vi "Reset WT300 Integrator.vi"(8 "error in (no error)":errorcluster, 11 "VISA resource name":refnum<visa-resource-name>) -> (0 "error out":errorcluster, 3 "VISA resource name out":refnum<visa-resource-name>)   [LabVIEW 2019, in "Yokogawa WT300 Series.lvlib"]
uses:
  Yokogawa WT300 Series.lvlib
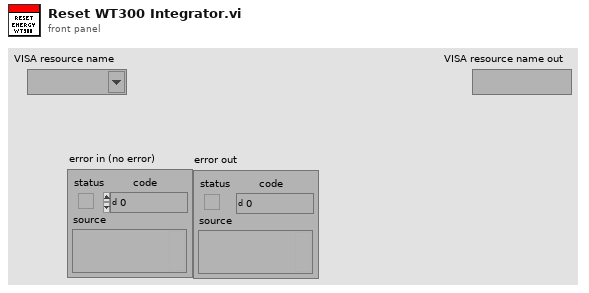
[diagram p1: front panel]
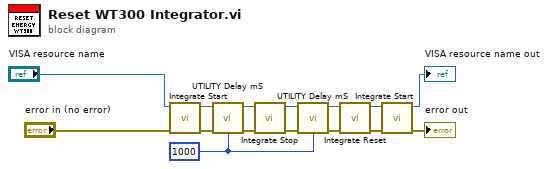
[diagram p0: block diagram]
diagram:
  w13 = u32 1000 ("milliseconds to wait")
  n1 = call "Integrate Start.vi"("error in (no error)"="error in (no error)", "VISA resource name"="VISA resource name") -> ("error out"=w7:errorcluster, "VISA resource name out"=w9:refnum<visa-resource-name>)  [unwired: 8 in]
  n2 = call "UTILITY Delay mS.vi"("Error In"=w7, "milliseconds to wait"=w13) -> ("Error Out"=w8:errorcluster)  [unwired: 13 in]
  n3 = call "Integrate Stop.vi"("error in (no error)"=w8, "VISA resource name"=w9) -> ("error out"=w11:errorcluster, "VISA resource name out"=w10:refnum<visa-resource-name>)  [unwired: 8 in]
  n4 = call "UTILITY Delay mS.vi"("Error In"=w11, "milliseconds to wait"=w13) -> ("Error Out"=w12:errorcluster)  [unwired: 13 in]
  n5 = call "Integrate Reset.vi"("error in (no error)"=w12, "VISA resource name"=w10) -> ("error out"=w3:errorcluster, "VISA resource name out"=w4:refnum<visa-resource-name>)  [unwired: 8 in]
  n6 = call "Integrate Start.vi"("error in (no error)"=w3, "VISA resource name"=w4) -> ("error out"=→"error out":errorcluster, "VISA resource name out"=→"VISA resource name out":refnum<visa-resource-name>)  [unwired: 8 in]
